vi "Ex_2.vi"() -> (3 "Waveform Graph 2":waveform(dbl)(graph))   [LabVIEW 2020]
uses:
  <vilib>/measure/NI_MABase.lvlib
panel:
  out "Fs":dbl format="%#_13g"
  out "Nyquist Equation":string
  out "Cycle of signals":i32
  in  "stop":bool
  in  "Amplitude  noise 2":dbl(knob)=1.0 min=0.001 max=1.0 step=0.1 scale=0.001..1.0
  in  "Frequency 2":dbl(knob)=100.0 min=100.0 max=10000.0 step=10.0 scale=100.0..10000.0
  in  "Amplitude 2":dbl(knob)=1.0 min=0.1 max=10.0 step=0.1 scale=0.1..10.0
  in  "Phase 2":dbl(slide) min=0.0 max=360.0 step=5.0 scale=0.0..360.0
  in  "Signal type 2":T1(ring)
  in  "sampling info 2":cluster{"Fs":dbl, "#s":dbl}={"Fs"=1000.0, "#s"=1000.0} {"Fs" format="%.2p"}
  in  "Square wave duty cycle (%) 2":dbl=50.0 format="%0.2f"
  in  "Offset 2":dbl(slide)=0.005 min=0.005 max=5.0 step=0.1 scale=0.005..5.0
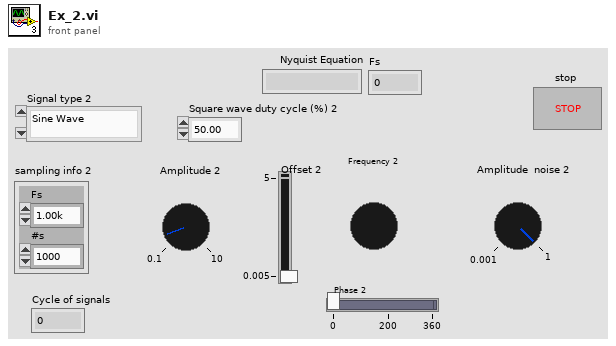
[diagram p1: front panel]
types:
  T1 = enum16{"Sine Wave", "Triangle Wave", "Square Wave", "Sawtooth Wave"}
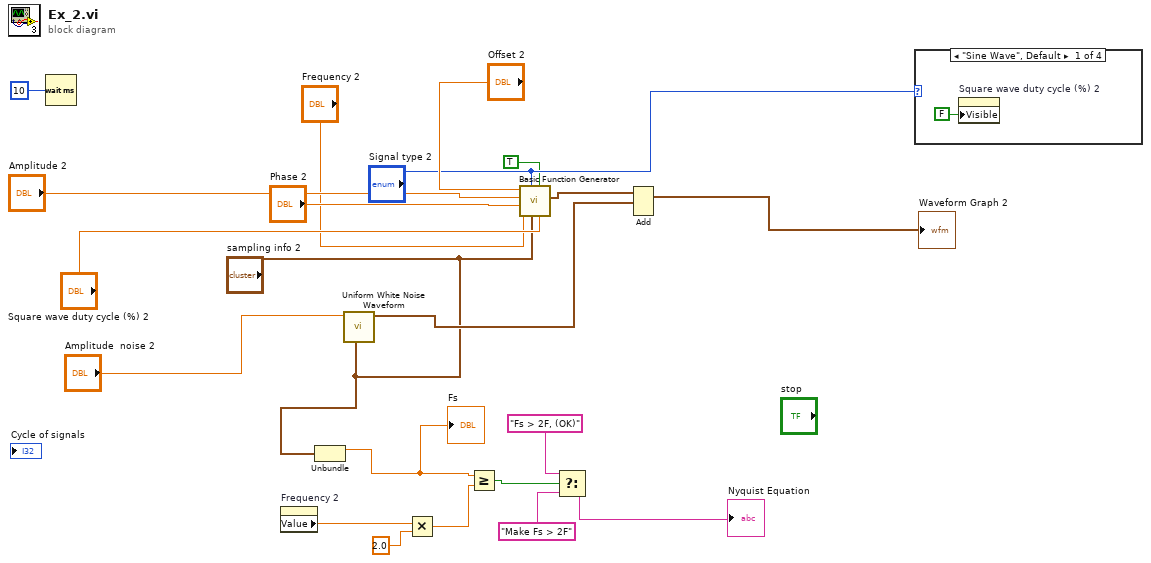
[diagram p0: block diagram]
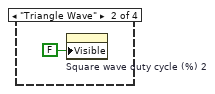
[diagram p2: hidden frame]
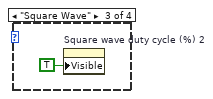
[diagram p3: hidden frame]
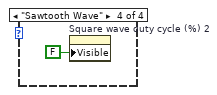
[diagram p4: hidden frame]
diagram:
  n1 = Wait (ms)(milliseconds to wait=10) -> ()  [unwired: 1 out]
  n2 = property on="Frequency 2" class="Knob (strict)"() -> ("Value"=w4:dbl)  [unwired: 2 in, 2 out]
  n3 = Unbundle("sampling info 2") -> ("Fs"=w2:dbl)  [unwired: 1 out]
  "Fs" <- w2
  n4 = call <vilib>:"Uniform White Noise Waveform.vi"("sampling info"="sampling info 2", "amplitude"="Amplitude  noise 2") -> ("signal out"=w13:waveform(dbl))  [unwired: 8 in, 1 out]
  n5 = Multiply(x=w4, y=2.0) -> (x*y=w6:dbl)
  n6 = Greater Or Equal?(x=w2, y=w6) -> (x >= y?=w8:bool)
  n7 = call <vilib>:"Basic Function Generator.vi"("offset"="Offset 2", "square wave duty cycle (%)"="Square wave duty cycle (%) 2", "reset signal"=TRUE, "sampling info"="sampling info 2", "signal type"="Signal type 2", "phase"="Phase 2", "amplitude"="Amplitude 2", "frequency"="Frequency 2") -> ("signal out"=w14:waveform(dbl))  [unwired: 1 in, 2 out]
  n8 = Select(t="Fs > 2F, (OK)", s=w8, f="Make Fs > 2F") -> (s? t:f=→"Nyquist Equation":string)
  n9 = Add(1:w13, 2:w14) -> (0:→"Waveform Graph 2":waveform(dbl))  [unwired: 1 in, 1 out]
  n10 = case shown="\"Sine Wave\", Default" "Signal type 2" {
    frame "Sine Wave", Default {
      n11 = property on="Square wave duty cycle (%) 2" class="DigNum (strict)"("Visible"=FALSE) -> ()  [unwired: 2 in, 2 out]
    }
    frame "Triangle Wave" {
      n12 = property on="Square wave duty cycle (%) 2" class="DigNum (strict)"("Visible"=FALSE) -> ()  [unwired: 2 in, 2 out]
    }
    frame "Square Wave" {
      n13 = property on="Square wave duty cycle (%) 2" class="DigNum (strict)"("Visible"=TRUE) -> ()  [unwired: 2 in, 2 out]
    }
    frame "Sawtooth Wave" {
      n14 = property on="Square wave duty cycle (%) 2" class="DigNum (strict)"("Visible"=FALSE) -> ()  [unwired: 2 in, 2 out]
    }
  }
